vi "Get File List.vi"(8 "error in (no error)":errorcluster, 9 "Connection Name":string, 11 "Remote Path":string) -> (0 "error out":errorcluster, 2 "File List":string, 3 "Return String":string)   [LabVIEW 2019, in "LabSFTP.lvlib"]
doc: "<License>This software is distributed under the BSD 3-Clause License. For the full license please see license.txt or visit www.labvolution.com/license</License>"
uses:
  LabSFTP.lvlib
  FGV State..enum.ctl
  C:/_Code/Development/Sub-Zero Functional Test/standard hardware/Universal Robots/UR LabVIEW Interface/LabSSH Library/References/LabSFTP.dll
  References/LabSFTP.dll
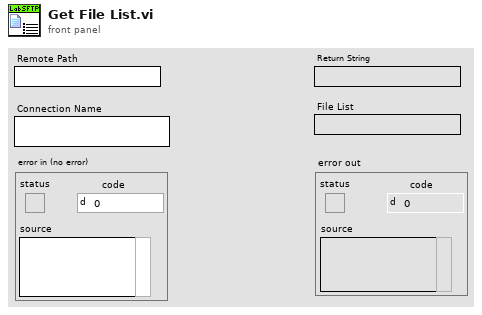
[diagram p1: front panel]
types:
  T1 = typedef "LabSFTP.lvlib/FGV State..enum.ctl" = enum16{"GET", "SET"}
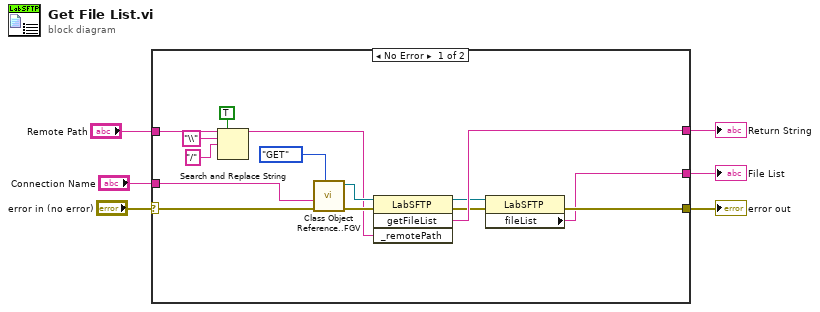
[diagram p0: block diagram]
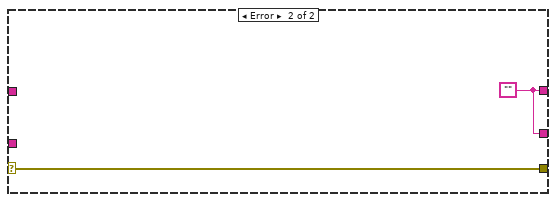
[diagram p2: hidden frame]
diagram:
  n1 = case shown="No Error" "error in (no error)" {
    selector: "error in (no error)" -> [w17 w23]
    tunnel: [w15 w23] -> w5
    tunnel: [w19 w22] -> w4
    tunnel: [w13 w22] -> w3
    tunnel: "Remote Path" -> [w9 _]
    tunnel: "Connection Name" -> [w7 _]
    frame No Error {
      n2 = Search and Replace String(replace all?=TRUE ("replace all? (F)"), input string=w9, search string="\\", replace string="/" ("replace string (\"\")")) -> (result string=w8:string)  [unwired: 4 in, 3 out]
      n3 = call "Class Object Reference..FGV.vi"("FGV State"=FGV_State..enum."GET", "error in (no error)"=w17, "Connection Name"=w7) -> ("error out"=w20:errorcluster, "LabSFTP ref out"=w21:refnum<k24>)  [unwired: 7 in]
      n4 = invoke class="LabSFTP" method="getFileList"(reference=w21, error in=w20, "_remotePath"=w8) -> (reference out=w14:refnum<k24>, error out=w18:errorcluster, "getFileList"=w19:string)  [unwired: 1 in, 1 out]
      n5 = property class="LabSFTP"(reference=w14, error in=w18) -> (error out=w15:errorcluster, "fileList"=w13:string)  [unwired: 1 out]
    }
    frame Error {
      w22 = ""
    }
  }
  "error out" <- w5
  "Return String" <- w4
  "File List" <- w3
